vi "PicowattAVS47_Manage_Monitor.vi"(2 "System Monitor Variables (in)":T1, 3 "Global Status (in)":T2 {"AVS Excitation" items=["no Exc", "3uV", "10uV", "30uV", "100uV", "300uV", "1mV", "3mV"]}, 4 "Command (in)":T2 {"AVS Excitation" items=["no Exc", "3uV", "10uV", "30uV", "100uV", "300uV", "1mV", "3mV"]}, 5 "Queue (in)":refnum<queue>) -> (0 "System Monitor Variables (out)":T1, 1 "Monitor (out)":T2 {"AVS Excitation" items=["no Exc", "3uV", "10uV", "30uV", "100uV", "300uV", "1mV", "3mV"]})   [LabVIEW 2019]
uses:
  PicowattAVS47/PicowattAVS47-Cluster.ctl
  Global/Global Variables/System Monitor Cluster.ctl
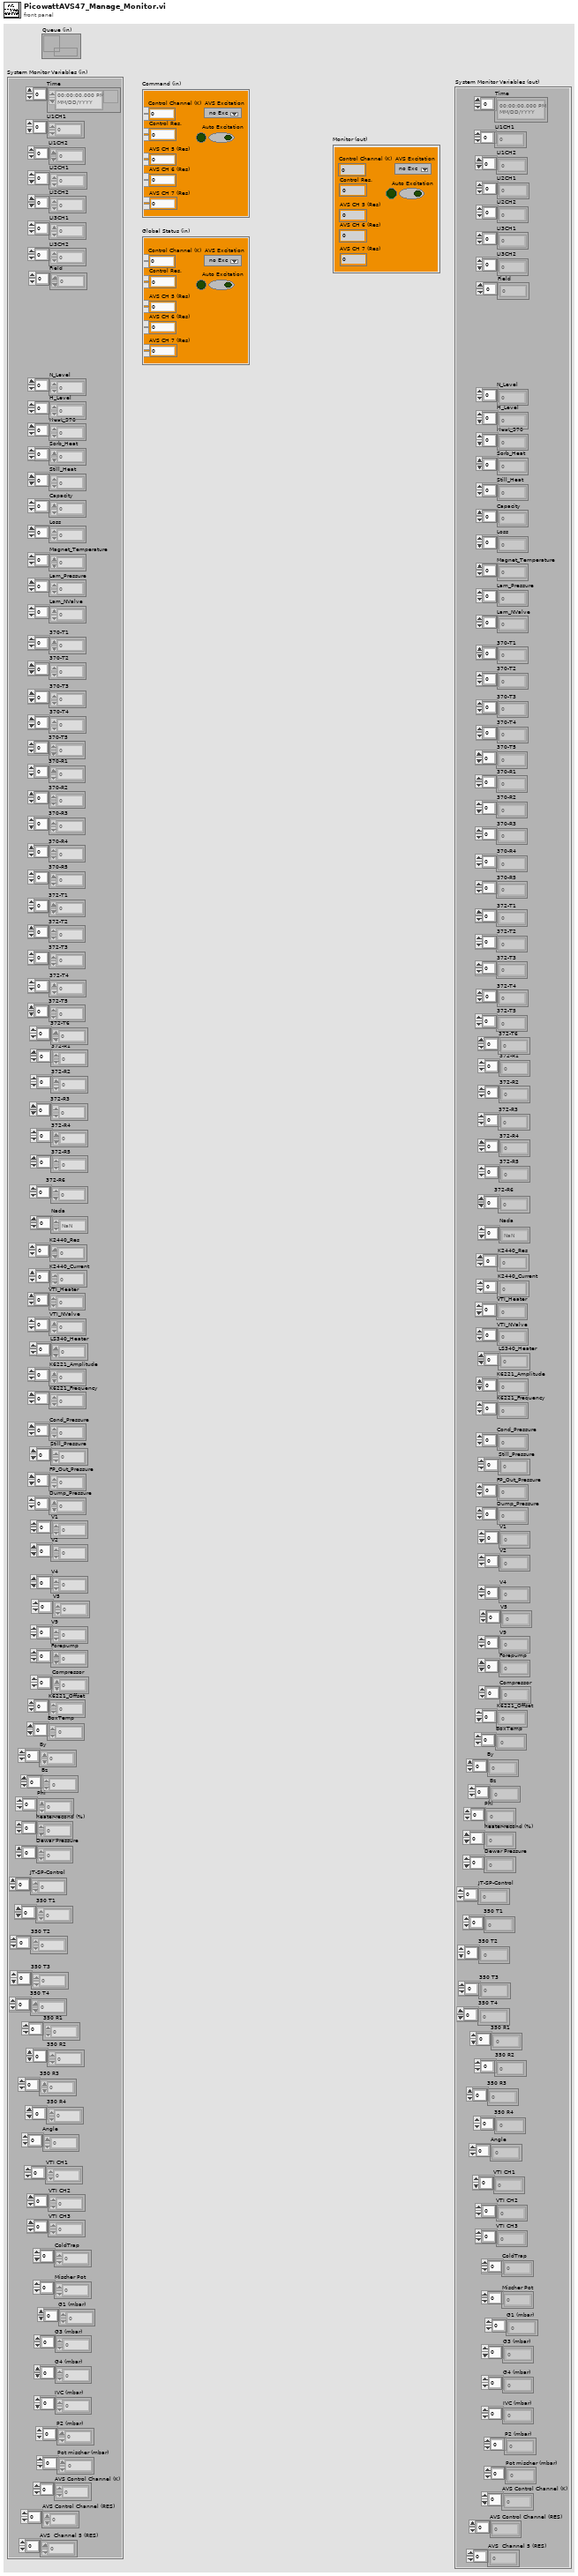
[diagram p1: front panel]
types:
  T1 = typedef "System Monitor Cluster.ctl" = cluster{"Time":timestamp[], "LI1CH1":dbl[], "LI1CH2":dbl[], "LI2CH1":dbl[], "LI2CH2":dbl[], "LI3CH1":dbl[], "LI3CH2":dbl[], "Field":dbl[], "N_Level":dbl[], "H_Level":dbl[], "Heat_370":dbl[], "Sorb_Heat":dbl[], "Still_Heat":dbl[], "Capacity":dbl[], "Loss":dbl[], "Magnet_Temperature":dbl[], "Lam_Pressure":dbl[], "Lam_NValve":dbl[], "370-T1":dbl[], "370-T2":dbl[], "370-T3":dbl[], "370-T4":dbl[], "370-T5":dbl[], "370-R1":dbl[], "370-R2":dbl[], "370-R3":dbl[], "370-R4":dbl[], "370-R5":dbl[], "372-T1":dbl[], "372-T2":dbl[], "372-T3":dbl[], "372-T4":dbl[], "372-T5":dbl[], "372-T6":dbl[], "372-R1":dbl[], "372-R2":dbl[], "372-R3":dbl[], "372-R4":dbl[], "372-R5":dbl[], "372-R6":dbl[], "Nada":dbl[], "K2440_Res":dbl[], "K2440_Current":dbl[], "VTI_Heater":dbl[], "VTI_NValve":dbl[], "LS340_Heater":dbl[], "K6221_Amplitude":dbl[], "K6221_Frequency":dbl[], "Cond_Pressure":dbl[], "Still_Pressure":dbl[], "FP_Out_Pressure":dbl[], "Dump_Pressure":dbl[], "V1":dbl[], "V2":dbl[], "V4":dbl[], "V5":dbl[], "V9":dbl[], "Forepump":dbl[], "Compressor":dbl[], "K6221_Offset":dbl[], "BoxTemp":dbl[], "By":dbl[], "Bz":dbl[], "Phi":dbl[], "heater-recond (%)":dbl[], "Dewar Pressure ":dbl[], "JT-SP-Control":dbl[], "350 T1":dbl[], "350 T2":dbl[], "350 T3":dbl[], "350 T4":dbl[], "350 R1":dbl[], "350 R2":dbl[], "350 R3":dbl[], "350 R4":dbl[], "Angle":dbl[], "VTI CH1":dbl[], "VTI CH2":dbl[], "VTI CH3":dbl[], "ColdTrap":dbl[], "Mischer Pot":dbl[], "G1 (mbar)":dbl[], "G3 (mbar) ":dbl[], "G4 (mbar)":dbl[], "IVC (mbar)":dbl[], "P2 (mbar) ":dbl[], "Pot mischer (mbar)":dbl[], "AVS Control Channel (K)":dbl[], "AVS Control Channel (RES)":dbl[], "AVS  Channel 5 (RES) ":dbl[]}
  T2 = typedef "PicowattAVS47-Cluster.ctl" = cluster{"Control Channel (K)":dbl, "AVS CH 5 (Res)":dbl, "AVS CH 6 (Res) ":dbl, "AVS CH 7 (Res) ":dbl, "Control Res.":dbl, "Auto Excitation":bool, "Auto activatet":bool, "AVS Excitation":i16}
  T3 = typedef "AVS-Control-Cluster.ctl" = cluster{"AVS Excitation":i16, "Auto Excitation":bool}
  T4 = typedef "AVS47-Status-Cluster.ctl" = cluster{"Control Channel (K)":dbl, "AVS CH 5 (Res)":dbl, "AVS CH 6 (Res) ":dbl, "AVS CH 7 (Res) ":dbl, "Control Res.":dbl, "Auto Exc. act":bool}
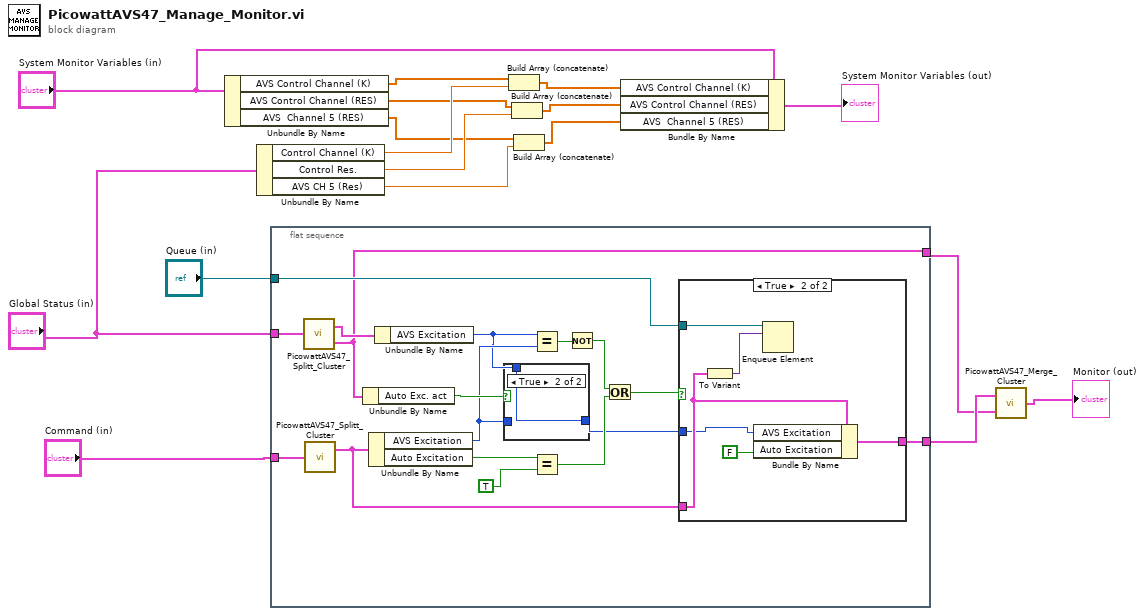
[diagram p0: block diagram]
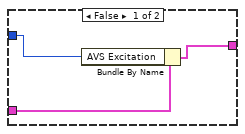
[diagram p3: hidden frame]
diagram:
  n1 = Unbundle By Name("System Monitor Variables (in)") -> ("AVS Control Channel (K)"=w16:dbl[], "AVS Control Channel (RES)"=w14:dbl[], "AVS  Channel 5 (RES)"=w12:dbl[])
  n2 = Unbundle By Name("Global Status (in)") -> ("Control Channel (K)"=w15:dbl, "Control Res."=w13:dbl, "AVS CH 5 (Res)"=w11:dbl)
  n3 = flat-sequence {
    tunnel: "Global Status (in)" -> [w34]
    tunnel: "Command (in)" -> [w33]
    tunnel: "Queue (in)" -> [w26]
    tunnel: [w25] -> w3
    tunnel: [w22] -> w2
    frame #0 {
      n4 = call "PicowattAVS47_Splitt_Cluster.vi"("Picowatt AVS47/TS530 Cluster"=w34) -> ("AVS47 Control Cluster"=w24:T3, "AVS47 Status Cluster"=w22:T4)
      n5 = call "PicowattAVS47_Splitt_Cluster.vi"("Picowatt AVS47/TS530 Cluster"=w33) -> ("AVS47 Control Cluster"=w23:T3)  [unwired: 1 out]
      n6 = Unbundle By Name(w22) -> ("Auto Exc. act"=w21:bool)
      n7 = Unbundle By Name(w23) -> ("AVS Excitation"=w20:i16, "Auto Excitation"=w32:bool)
      n8 = Unbundle By Name(w24) -> ("AVS Excitation"=w18:i16)
      n9 = case shown="True" w21 {
        tunnel: [w35 w36] -> w19
        tunnel: w20 -> [w35 _]
        tunnel: w18 -> [_ w36]
        frame False {
        }
        frame True {
        }
      }
      n10 = Equal?(x=w18, y=w20) -> (x = y?=w30:bool)
      n11 = Equal?(x=w32, y=TRUE) -> (x = y?=w28:bool)
      n12 = Not(x=w30) -> (.not. x?=w29:bool)
      n13 = Or(x=w29, y=w28) -> (x .or. y?=w27:bool)
      n14 = case shown="True" w27 {
        tunnel: w23 -> [w39 w43]
        tunnel: w26 -> [_ w45]
        tunnel: [w38 w41] -> w25
        tunnel: w19 -> [w37 w40]
        frame False {
          n15 = Bundle By Name(cluster=w39, "AVS Excitation"=w37) -> (w38:T3)
        }
        frame True {
          n16 = To Variant(anything=w43) -> (Variant=w44:variant)
          n17 = Bundle By Name(cluster=w43, "AVS Excitation"=w40, "Auto Excitation"=FALSE) -> (w41:T3)
          n18 = Enqueue Element(queue=w45, element=w44) -> ()  [unwired: 2 in, 3 out]
        }
      }
    }
  }
  n19 = Build Array (concatenate)(w16, w15) -> (w9:dbl[])
  n20 = Build Array (concatenate)(w14, w13) -> (w8:dbl[])
  n21 = Build Array (concatenate)(w12, w11) -> (w7:dbl[])
  n22 = Bundle By Name(cluster="System Monitor Variables (in)", "AVS Control Channel (K)"=w9, "AVS Control Channel (RES)"=w8, "AVS  Channel 5 (RES)"=w7) -> (→"System Monitor Variables (out)":T1)
  n23 = call "PicowattAVS47_Merge_Cluster.vi"("AVS47 Status Cluster"=w2, "AVS47 Control Cluster"=w3) -> ("Picowatt AVS47/TS530 Cluster"=→"Monitor (out)":T2)
